vi "Command Loop - Apply Config.vi"(8 "error in":errorcluster, 10 "Data":u8[](array[numeric]), 11 "Queue Refs in":variant) -> (0 "error out":errorcluster, 2 "Response":string, 3 "Queue Refs out":variant)   [LabVIEW 2026, in "Runtime Configuration Support Inline Async Example Custom Device Engine.lvlib"]
uses:
  Runtime Configuration Support Inline Async Example Custom Device Engine.lvlib
  Shared/Reconfigured.Settings.ctl
  Shared/Compiled.Settings.ctl
  <vilib>/NI VeriStand/Custom Device API/Block Data Reference.ctl
  <vilib>/NI VeriStand/Custom Device API/Data Reference.ctl
  <vilib>/NI VeriStand/Custom Device API/Custom Device API.lvlib
  Shared/Runtime Configuration Support Inline Async Example Custom Device Shared.lvlib
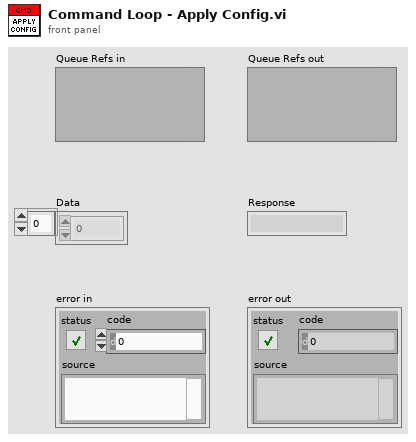
[diagram p1: front panel]
types:
  T1 = typedef "Runtime Configuration Support Inline Async Example Custom Device Shared.lvlib/Reconfigured.Settings.ctl" = cluster{"Compiled.Settings":T2, "Compiled Inline Async Settings":cluster{"Read":cluster{"Refs":T3[], "Values":dbl[]}[], "Write":cluster{"Refs":T3[], "Values":dbl[]}[], "ReadWrite":cluster{"Refs":T4[], "Values":dbl[], "Reset Values":dbl[]}[], "LUT":variant}, "Response Ref":refnum<queue>}
  T2 = typedef "Runtime Configuration Support Inline Async Example Custom Device Shared.lvlib/Compiled.Settings.ctl" = cluster{"Name":string, "Async Init Timeout":u16, "Inport SignalIDs":i32[], "Outport SignalIDs":i32[], "Inport Values":dbl[], "Outport Values":dbl[], "Dynamic Config Status":bool, "Device Error":errorcluster}
  T3 = typedef "Custom Device API.lvlib/Block Data Reference.ctl" = cluster{"Data Reference":T4, "Offset":u64, "Length":u64}
  T4 = typedef "Custom Device API.lvlib/Data Reference.ctl" = i32
  T5 = cluster{"Dynamic Config Status":bool, "Error":errorcluster}
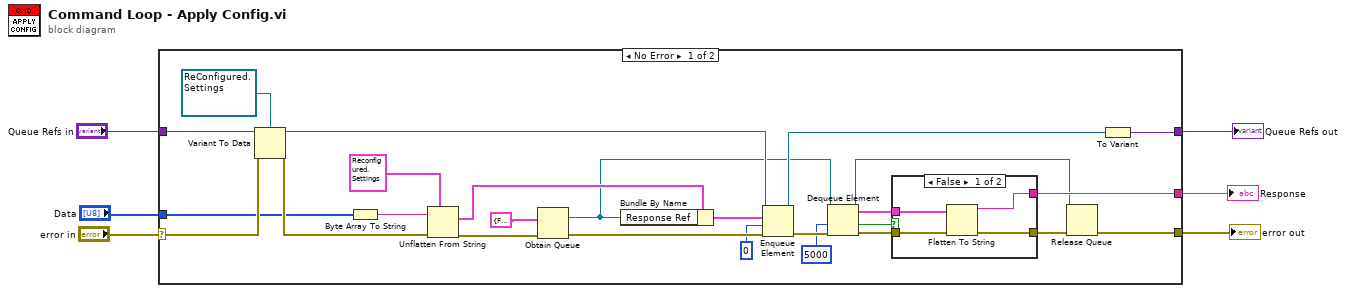
[diagram p0: block diagram]
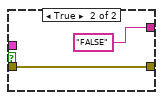
[diagram p2: hidden frame]
diagram:
  n1 = case shown="No Error" "error in" {
    selector: "error in" -> [w31 w40]
    tunnel: [w32 w40] -> w6
    tunnel: "Data" -> [w24 _]
    tunnel: [w23 _] -> w3
    tunnel: "Queue Refs in" -> [w22 w39]
    tunnel: [w20 w39] -> w1
    frame No Error {
      n2 = Variant To Data(error in=w31, type=refnum<queue> refnum ("ReConfigured.Settings Ref"), Variant=w22) -> (data=w21:refnum<queue>, error out=w30:errorcluster)
      n3 = Byte Array To String(unsigned byte array=w24) -> (string=w18:string)
      n4 = Unflatten From String(type=T1 {"Compiled.Settings"={"Name"="", "Async Init Timeout"=0, "Inport SignalIDs"=[], "Outport SignalIDs"=[], "Inport Values"=[], "Outport Values"=[], "Dynamic Config Status"=FALSE, "Device Error"={"status"=FALSE, "code"=0, "source"=""}}, "Compiled Inline Async Settings"={"Read"=[], "Write"=[], "ReadWrite"=[], "LUT"=variant}, "Response Ref"=refnum} ("ReConfigured.Settings"), binary string=w18, error in (no error)=w30) -> (value=w15:T1, error out=w29:errorcluster)  [unwired: 2 in, 1 out]
      n5 = Obtain Queue(element data type=T5 {"Dynamic Config Status"=FALSE, "Error"={"status"=FALSE, "code"=0, "source"=""}}, error in (no error)=w29) -> (queue out=w10:refnum<queue>, error out=w28:errorcluster)  [unwired: 3 in, 1 out]
      n6 = Bundle By Name(cluster=w15, "Response Ref"=w10) -> (w8:T1)
      n7 = Enqueue Element(queue=w21, element=w8, timeout in ms (-1)=0, error in (no error)=w28) -> (queue out=w16:refnum<queue>, error out=w27:errorcluster)  [unwired: 1 out]
      n8 = Dequeue Element(queue=w10, timeout in ms (-1)=5000, error in (no error)=w27) -> (queue out=w11:refnum<queue>, element=w14:T5, timed out?=w13:bool, error out=w25:errorcluster)
      n9 = case shown="False" w13 {
        tunnel: w14 -> [w33 _]
        tunnel: [w34 "FALSE"] -> w23
        tunnel: w25 -> [w36 w38]
        tunnel: [w35 w38] -> w26
        frame False {
          n10 = Flatten To String(anything=w33, error in (no error)=w36) -> (data string=w34:string, error out=w35:errorcluster)  [unwired: 2 in, 1 out]
        }
        frame True {
        }
      }
      n11 = Release Queue(queue=w11, error in (no error)=w26) -> (error out=w32:errorcluster)  [unwired: 1 in, 2 out]
      n12 = To Variant(anything=w16) -> (Variant=w20:variant)
    }
    frame Error {
    }
  }
  "error out" <- w6
  "Response" <- w3
  "Queue Refs out" <- w1
